vi "sample_frequency.vi"() -> (0 "Sample frequency":dbl)   [LabVIEW 2013]
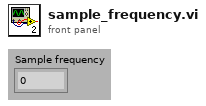
[diagram p1: front panel]
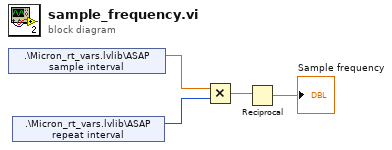
[diagram p0: block diagram]
diagram:
  n1 = shared-variable ".\\Micron_rt_vars.lvlib\\ASAP sample interval"() -> (w2:dbl)  [unwired: 2 out]
  n2 = shared-variable ".\\Micron_rt_vars.lvlib\\ASAP repeat interval"() -> (w1:i32)  [unwired: 2 out]
  n3 = Multiply(x=w2, y=w1) -> (x*y=w3:dbl)
  n4 = Reciprocal(x=w3) -> (1/x=→"Sample frequency":dbl)
